vi "4.7.vi"() -> ()   [LabVIEW 2017]
panel:
  out "猜测次数":dbl
  out "随机的数":u32
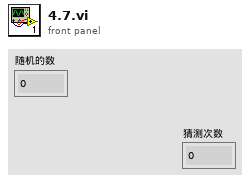
[diagram p1: front panel]
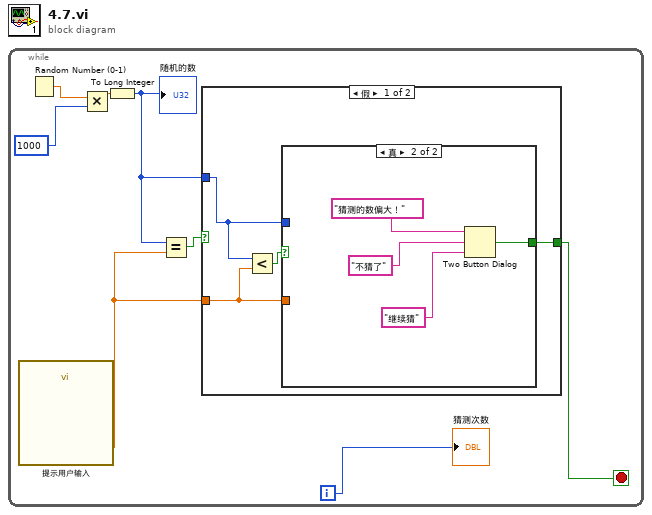
[diagram p0: block diagram]
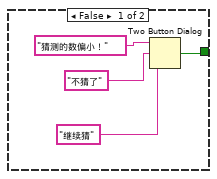
[diagram p2: hidden frame]
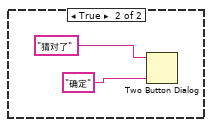
[diagram p3: hidden frame]
diagram:
  n1 = while {
    i -> [w6]
    stop <- w3 stop-if-true
    n2 = call "提示用户输入"() -> ("请在1-1000猜"=w5:dbl)  [unwired: 17 in, 2 out]
    n3 = Random Number (0-1)() -> (number: 0 to 1=w8:dbl)
    n4 = Multiply(x=w8, y=1000) -> (x*y=w2:dbl)
    n5 = To Long Integer(number=w2) -> (32bit integer=w1:i32)
    "随机的数" <- w1
    n6 = Equal?(x=w1, y=w5) -> (x = y?=w4:bool)
    n7 = case shown="假" w4 {
      tunnel: w5 -> [w9 _]
      tunnel: w1 -> [w10 _]
      tunnel: [w12 _] -> w3
      frame False {
        n8 = Less?(x=w10, y=w9) -> (x < y?=w11:bool)
        n9 = case shown="真" w11 {
          tunnel: [w13 w18] -> w12
          tunnel: w10 -> [_ _]
          tunnel: w9 -> [_ _]
          frame False {
            n10 = Two Button Dialog(message="猜测的数偏小！", 1:"继续猜", 2:"不猜了") -> (T button?=w13:bool)
          }
          frame True {
            n11 = Two Button Dialog(message="猜测的数偏大！", 1:"继续猜", 2:"不猜了") -> (T button?=w18:bool)
          }
        }
      }
      frame True {
        n12 = Two Button Dialog(message="猜对了", 1:"确定") -> ()  [unwired: 1 in, 1 out]
      }
    }
    "猜测次数" <- w6
  }
